vi "Condiciones_And_Or.vi"() -> ()   [LabVIEW 2013]
panel:
  in  "Seleccionar local":u16(ring) items=["Local 1", "Local 2", "Local 3"]
  out "A/C":bool
  out "NumeroPersonas":i32
  out "Temperatura":i32(slide) scale=0.0..60.0
  # "Debemos seleccionar el local, luego generar\nel numero de personas entre 1-50 y la temperatura\nentre 1-60.\nEl A/C se enciende de acuerdo a los siguientes casos:\n\nLocal              Condicion para encender el A/C\n\nLocal 1            Si la temperatura es mayor a 25 o el numero de empleados es mayor a 30.\nLocal 2            Si la temperatura es mayor a 28 o el numero de empleados es mayor a 35.\nLocal 3            Si la temperatura es mayor a 24 o el numero de empleados es mayor a 20."
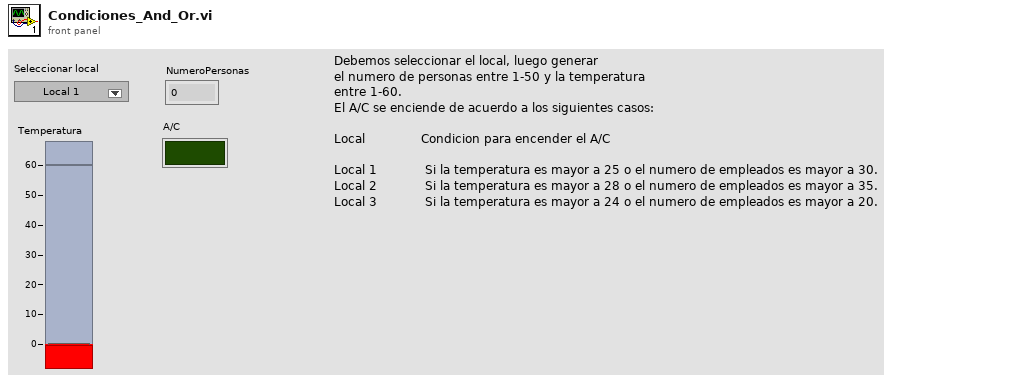
[diagram p1: front panel]
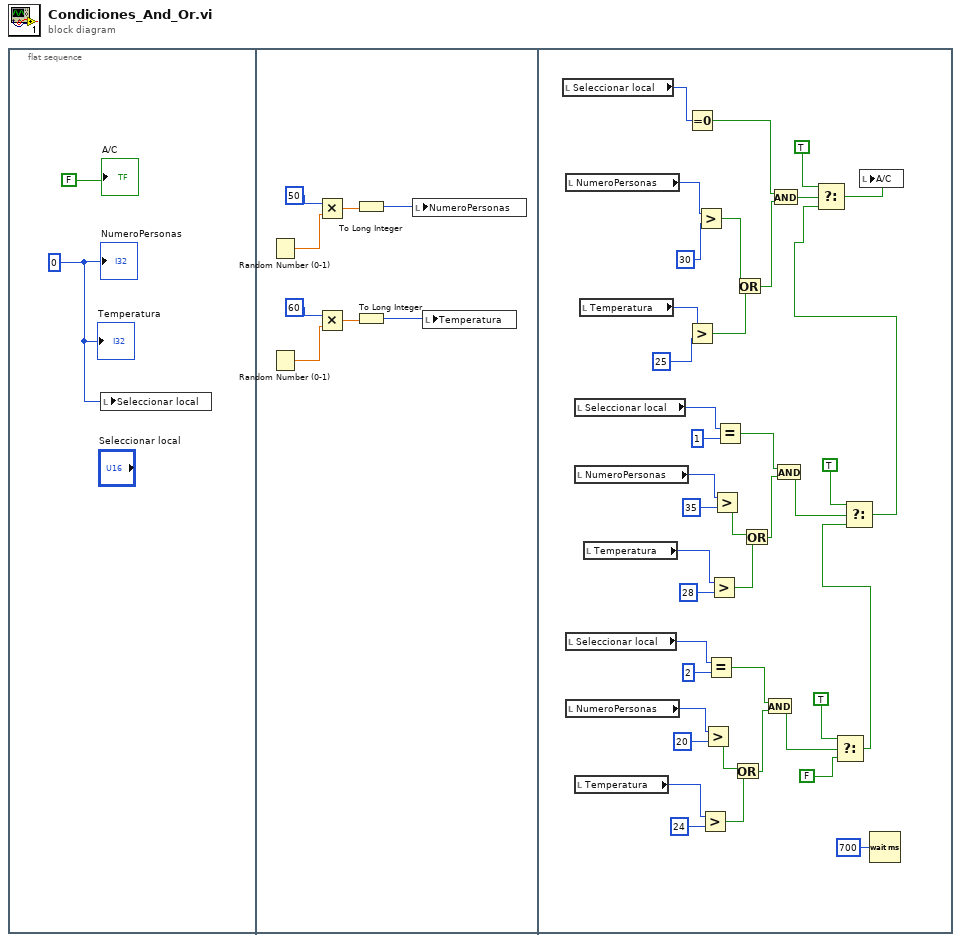
[diagram p0: block diagram]
diagram:
  n1 = flat-sequence {
    frame #0 {
      w1 = 0 ("NumeroPersonas")
      n2 = local write "Seleccionar local"(w1) -> ()
      "Temperatura" <- w1
      "NumeroPersonas" <- w1
      "A/C" <- FALSE
    }
    frame #1 {
      n3 = Random Number (0-1)() -> (number: 0 to 1=w8:dbl)
      n4 = Random Number (0-1)() -> (number: 0 to 1=w5:dbl)
      n5 = Multiply(x=50, y=w8) -> (x*y=w10:dbl)
      n6 = Multiply(x=60, y=w5) -> (x*y=w3:dbl)
      n7 = To Long Integer(number=w10) -> (32bit integer=w9:i32)
      n8 = To Long Integer(number=w3) -> (32bit integer=w4:i32)
      n9 = local write "NumeroPersonas"(w9) -> ()
      n10 = local write "Temperatura"(w4) -> ()
    }
    frame #2 {
      n11 = local read "Seleccionar local"() -> (w50:u16)
      n12 = local read "NumeroPersonas"() -> (w49:i32)
      n13 = local read "Seleccionar local"() -> (w14:u16)
      n14 = local read "NumeroPersonas"() -> (w17:i32)
      n15 = local read "Seleccionar local"() -> (w38:u16)
      n16 = local read "NumeroPersonas"() -> (w35:i32)
      n17 = local read "Temperatura"() -> (w19:i32)
      n18 = local read "Temperatura"() -> (w46:i32)
      n19 = local read "Temperatura"() -> (w33:i32)
      n20 = Equal To 0?(x=w50) -> (x = 0?=w42:bool)
      n21 = Greater?(x=w46, y=25) -> (0:w44:bool)
      n22 = Greater?(x=w49, y=30) -> (0:w45:bool)
      n23 = Greater?(x=w19, y=u16 24) -> (0:w21:bool)
      n24 = Greater?(x=w17, y=u16 20) -> (0:w20:bool)
      n25 = Equal?(x=w14, y=u16 2) -> (x = y?=w23:bool)
      n26 = Greater?(x=w33, y=u16 28) -> (0:w31:bool)
      n27 = Greater?(x=w35, y=u16 35) -> (0:w32:bool)
      n28 = Equal?(x=w38, y=u16 1) -> (x = y?=w29:bool)
      n29 = Or(x=w20, y=w21) -> (x .or. y?=w22:bool)
      n30 = Or(x=w45, y=w44) -> (x .or. y?=w43:bool)
      n31 = Or(x=w32, y=w31) -> (x .or. y?=w30:bool)
      n32 = And(x=w23, y=w22) -> (x .and. y?=w25:bool)
      n33 = And(x=w42, y=w43) -> (x .and. y?=w41:bool)
      n34 = And(x=w29, y=w30) -> (x .and. y?=w27:bool)
      n35 = Select(t=TRUE, s=w25, f=FALSE) -> (s? t:f=w12:bool)
      n36 = Select(t=TRUE, s=w27, f=w12) -> (s? t:f=w26:bool)
      n37 = Select(t=TRUE, s=w41, f=w26) -> (s? t:f=w39:bool)
      n38 = local write "A/C"(w39) -> ()
      n39 = Wait (ms)(milliseconds to wait=u32 700) -> ()  [unwired: 1 out]
    }
  }
